vi "Elmo reset.vi"(8 "에러 입력":errorcluster caption="에러 출력", 11 "Motor status":T1(ring)=enum."Snyc") -> (0 "에러 출력":errorcluster caption="error IO", 2 "status 1":u16, 3 "Status 0":u16)   [LabVIEW 2019]
uses:
  Elmo Status.ctl
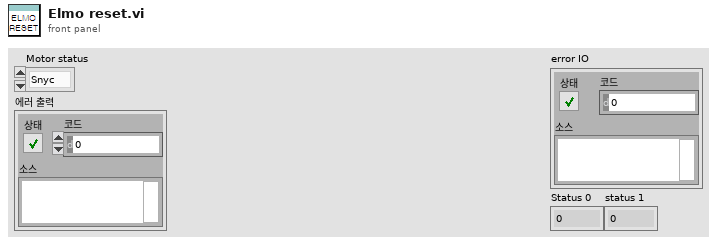
[diagram p1: front panel]
types:
  T1 = enum16{"Init", "ChkRdy", "Snyc", "Tuning", "Manual"}
  T2 = typedef "Elmo Status.ctl" = enum16{"Not ready to switch on", "Switch on disabled", "Ready to switch on", "Switch on", "Operation Enabled", "Quick stop active", "Fault reaction active", "Fault", "None"}
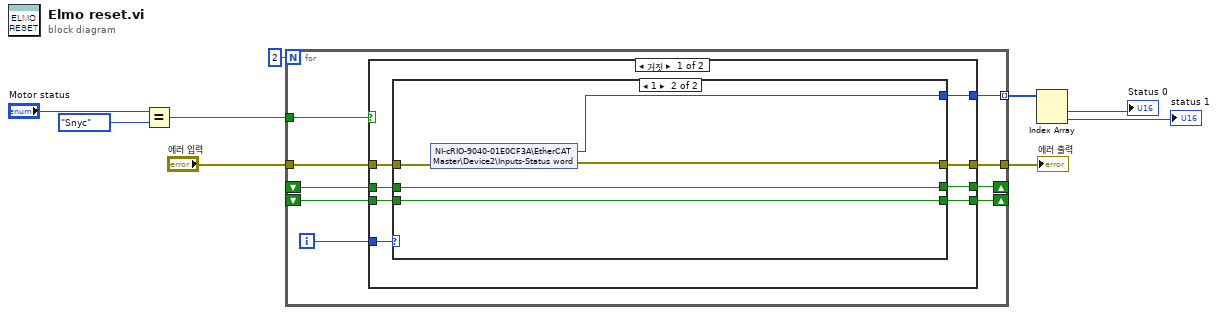
[diagram p0: block diagram]
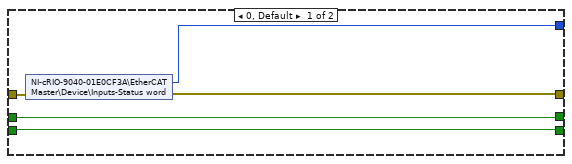
[diagram p2: hidden frame]
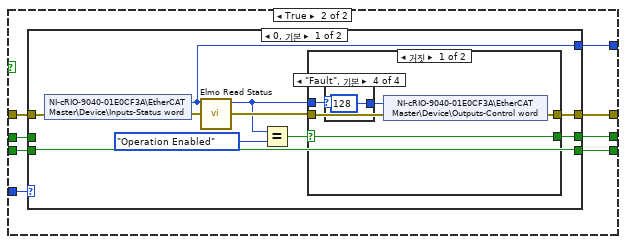
[diagram p3: hidden frame]
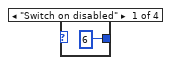
[diagram p4: hidden frame]
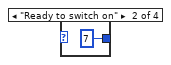
[diagram p5: hidden frame]
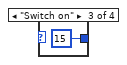
[diagram p6: hidden frame]
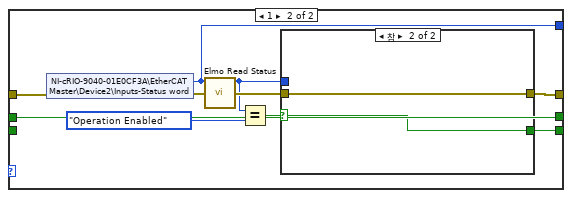
[diagram p8: hidden frame]
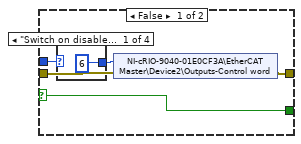
[diagram p9: hidden frame]
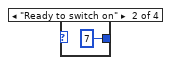
[diagram p10: hidden frame]
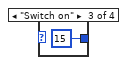
[diagram p11: hidden frame]
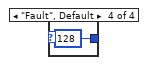
[diagram p12: hidden frame]
diagram:
  n1 = Equal?(x="Motor status", y=T1."Snyc") -> (x = y?=w4:bool)
  n2 = for {
    N: 2 -> [_]
    tunnel: "에러 입력" -> [w17]
    tunnel: [w16] -> w6
    shift-right: [w15] -> _
    shift-left: _ -> [w14]
    shift-right: [w13] -> _
    shift-left: _ -> [w12]
    tunnel: w4 -> [w11]
    tunnel: [w10] -> w3 mode=indexing
    i -> [w18]
    n3 = case shown="거짓" w11 {
      tunnel: w18 -> [w26 w44]
      tunnel: w17 -> [w19 w43]
      tunnel: [w21 w42] -> w16
      tunnel: [w23 w41] -> w15
      tunnel: w14 -> [w25 w40]
      tunnel: [w22 w39] -> w13
      tunnel: w12 -> [w24 w38]
      tunnel: [w20 w37] -> w10
      frame False {
        n4 = case shown="1" w26 {
          tunnel: w19 -> [w31 w36]
          tunnel: [w28 w32] -> w21
          tunnel: [w27 w35] -> w23
          tunnel: w25 -> [w27 w35]
          tunnel: [w30 w33] -> w22
          tunnel: w24 -> [w30 w33]
          tunnel: [w29 w34] -> w20
          frame 0, Default {
            n5 = shared-variable "NI-cRIO-9040-01E0CF3A\\EtherCAT Master\\Device\\Inputs-Status word"(error in=w31) -> (w29:u16, error out=w28:errorcluster)
          }
          frame 1 {
            n6 = shared-variable "NI-cRIO-9040-01E0CF3A\\EtherCAT Master\\Device2\\Inputs-Status word"(error in=w36) -> (w34:u16, error out=w32:errorcluster)
          }
        }
      }
      frame True {
        n7 = case shown="0, 기본" w44 {
          tunnel: w43 -> [w53 w73]
          tunnel: [w51 w71] -> w42
          tunnel: [w47 w66] -> w41
          tunnel: w40 -> [_ w66]
          tunnel: [w46 w67] -> w39
          tunnel: w38 -> [w46 _]
          tunnel: [w45 w65] -> w37
          frame 0, Default {
            n8 = shared-variable "NI-cRIO-9040-01E0CF3A\\EtherCAT Master\\Device\\Inputs-Status word"(error in=w53) -> (w45:u16, error out=w52:errorcluster)
            n9 = call "Elmo Read Status.vi"("State Word"=w45) -> ("Elmo State"=w49:T2)  [unwired: 7 in, 3 out]
            n10 = Equal?(x=w49, y=Elmo_Status."Operation Enabled" ("Elmo State")) -> (x = y?=w50:bool)
            n11 = case shown="거짓" w50 {
              selector: w50 -> [w56 w63]
              tunnel: w52 -> [w58 w64]
              tunnel: [w57 w64] -> w51
              tunnel: w49 -> [w55 _]
              tunnel: [w56 w63] -> w47
              frame False {
                n12 = case shown="\"Fault\", 기본" w55 {
                  tunnel: [u16 6 u16 7 u16 15 u16 128] -> w54
                  frame "Switch on disabled" {
                  }
                  frame "Ready to switch on" {
                  }
                  frame "Switch on" {
                  }
                  frame "Fault", Default {
                  }
                }
                n13 = shared-variable "NI-cRIO-9040-01E0CF3A\\EtherCAT Master\\Device\\Outputs-Control word"(w54, error in=w58) -> (error out=w57:errorcluster)
              }
              frame True {
              }
            }
          }
          frame 1 {
            n14 = shared-variable "NI-cRIO-9040-01E0CF3A\\EtherCAT Master\\Device2\\Inputs-Status word"(error in=w73) -> (w65:u16, error out=w72:errorcluster)
            n15 = call "Elmo Read Status.vi"("State Word"=w65) -> ("Elmo State"=w70:T2)  [unwired: 7 in, 3 out]
            n16 = Equal?(x=w70, y=Elmo_Status."Operation Enabled" ("Elmo State")) -> (x = y?=w69:bool)
            n17 = case shown="참" w69 {
              selector: w69 -> [w78 w83]
              tunnel: w72 -> [w75 w84]
              tunnel: [w74 w84] -> w71
              tunnel: w70 -> [w77 _]
              tunnel: [w78 w83] -> w67
              frame False {
                n18 = case shown="\"Switch on disabled\"" w77 {
                  tunnel: [u16 6 u16 7 u16 15 u16 128] -> w76
                  frame "Switch on disabled" {
                  }
                  frame "Ready to switch on" {
                  }
                  frame "Switch on" {
                  }
                  frame "Fault", Default {
                  }
                }
                n19 = shared-variable "NI-cRIO-9040-01E0CF3A\\EtherCAT Master\\Device2\\Outputs-Control word"(w76, error in=w75) -> (error out=w74:errorcluster)
              }
              frame True {
              }
            }
          }
        }
      }
    }
  }
  "에러 출력" <- w6
  n20 = Index Array(array=w3) -> (element #1=→"Status 0":u16, element #2=→"status 1":u16)  [unwired: 2 in]
